vi "pointB.vi"() -> ()   [LabVIEW 2011]
panel:
  out "data out":dbl[][](array[numeric])
  out "Numeric":i32
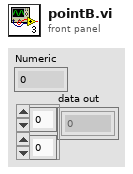
[diagram p1: front panel]
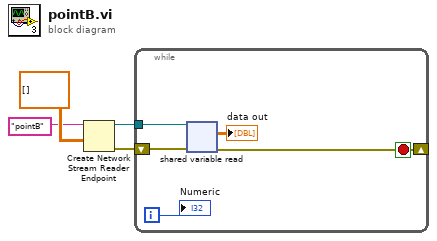
[diagram p0: block diagram]
diagram:
  n1 = Create Network Stream Reader Endpoint(9:dbl[][] [], 11:"pointB" ("writer name")) -> (0:w2:errorcluster, 3:w1:refnum<k21>)  [unwired: 4 in]
  n2 = while {
    tunnel: w1 -> [w7]
    shift-right: [w5] -> _
    shift-left: w2 -> [w8]
    i -> [w9]
    stop <- w5 stop-if-true
    n3 = shared-variable-read(w7, w8) -> (w5:errorcluster, →"data out":dbl[][])  [unwired: 1 in, 2 out]
    "Numeric" <- w9
  }
